vi "RGB to Color.vi"(1 "B":u8, 2 "G":u8, 3 "R":u8) -> (0 "Color":u32(colorbox))   [LabVIEW 2020]
doc: "Converts a red, green, and blue value from 0 to 255 to the corresponding RGB color."
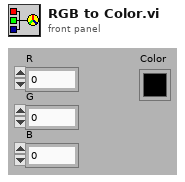
[diagram p1: front panel]
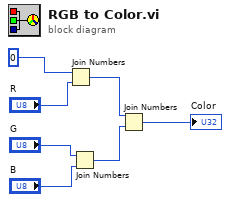
[diagram p0: block diagram]
diagram:
  n1 = Join Numbers(hi=u8 0, lo="R") -> ((hi.lo)=w3:u16)
  n2 = Join Numbers(hi="G", lo="B") -> ((hi.lo)=w2:u16)
  n3 = Join Numbers(hi=w3, lo=w2) -> ((hi.lo)=→"Color":u32)
